vi "le fpga.vi"() -> ()   [LabVIEW 2016]
uses:
  <vilib>/LabVIEW Targets/FPGA/cRIO/shared/nicrio_ModuleControls/nicrio_cRIO-9871_BaudRateEnum.ctl
  <vilib>/LabVIEW Targets/FPGA/cRIO/shared/nicrio_ModuleControls/nicrio_cRIO-9871_ParityEnum.ctl
  <vilib>/LabVIEW Targets/FPGA/cRIO/shared/nicrio_ModuleControls/nicrio_cRIO-9871_StopBitsEnum.ctl
  <vilib>/LabVIEW Targets/FPGA/cRIO/shared/nicrio_ModuleControls/nicrio_cRIO-9871_DataBitsEnum.ctl
  <vilib>/Platform/TimedLoop/XDataNode/timing_clust.ctl
  <vilib>/Platform/TimedLoop/XDataNode/nitl_modes.ctl
  <vilib>/Platform/TimedLoop/XDataNode/wakeup.ctl
  <vilib>/rvi/FXPMathLib/basic elements/FxpIntAccumulator/subVIs/nifxpmath_IntAccumulator_SimConfig.ctl
  <vilib>/rvi/Emulation/niFpgaGetClockAttributes.vi
  <vilib>/rvi/Emulation/niFpgaSctlEmulationGetInTimedLoop.vi
  <vilib>/rvi/Emulation/niFpgaEmulationReportErrorSimple.vi
  <vilib>/rvi/eio/common/nirviEmuTemplateMethod_errors.vi
  <vilib>/rvi/Emulation/niFpgaCriticalErrorInLSC.vi
  <vilib>/rvi/Analysis/common/codeGenErrors/XNode/niFpgaXNodeCodeGenErrorHandle.vi
  <vilib>/rvi/FXPMathLib/basic elements/FxpIntAccumulator/simVIs/DllFxpIntAccumulator_sub.vi
  <vilib>/rvi/eio/common/nirviEmuTemplatePropertySet_noerrors.vi
  <vilib>/eio/EIONode/EIONode.xnode
  <vilib>/eio/EIOMethodNode/EIOMethodNode.xnode
  <vilib>/rvi/Analysis/measure/dc-rms/XNode/niFpgaDC-RMS.xnode
  <vilib>/Platform/TimedLoop/XDataNode/XDataNode.xnode
  <vilib>/rvi/FXPMathLib/basic elements/FxpIntAccumulator/XNode/nifxpmath_IntAccumulator.xnode
  <vilib>/rvi/FXPMathLib/FxpMul/XNode/nifxpmath_Multiplier.xnode
  <vilib>/eio/EIOPropertyNode/EIOPropertyNode.xnode
  <vilib>/Platform/TimedLoop/XDataNode/XDNodeRunTimeDep.lvlib
  <vilib>/rvi/FXPMathLib/sim/FxpSim.dll
  <vilib>/rvi/eio/common/nirviEmuTemplatePropertyGet_errors.vi
  <vilib>/rvi/eio/common/nirviEmuTemplatePropertyGet_noerrors.vi
  <vilib>/rvi/eio/common/nirviEmuTemplatePropertySet_errors.vi
panel:
  out "Time since repurge":u8[](array[numeric])
  out "1st stage temp(k)":u8[](array[numeric])
  out "2nd stage":u8[](array[numeric])
  out "Time on":u8[](array[numeric])
  out "Pump On":u8[](array[numeric])
  out "Ion gauge 6":u8[](array[numeric])
  out "Convectron 6":u8[](array[numeric])
  out "Convectron 5":u8[](array[numeric])
  out "Ion gauge 5":u8[](array[numeric])
  out "Analog input  2":fxp<+/-,26,5>[](array[numeric]) format="%.23g"
  in  "analog output 2":fxp<+/-,64,32>[](array[numeric])=[0.0, 0.0, 0.0, 0.0, 0.0, 0.0, 0.0]
  out "Digital readback":bool[](array[boolean])
  in  "inj image ap":bool
  in  "LE waist ap":bool
  in  "LE Waist FC":bool
  in  "ATTEN":bool
  in  "inj image  FC":bool
  in  "LE FC":bool
  out "Ion gauge 4":u8[](array[numeric])
  out "Convectron 4":u8[](array[numeric])
  out "Convectron 3":u8[](array[numeric])
  out "Ion gauge 3":u8[](array[numeric])
  in  "analog output":fxp<+/-,64,32>[](array[numeric])=[0.0, 0.0, 0.0, 0.0, 0.0, 0.0, 0.0]
  out "Analog input":fxp<+/-,26,5>[](array[numeric]) format="%.23g"
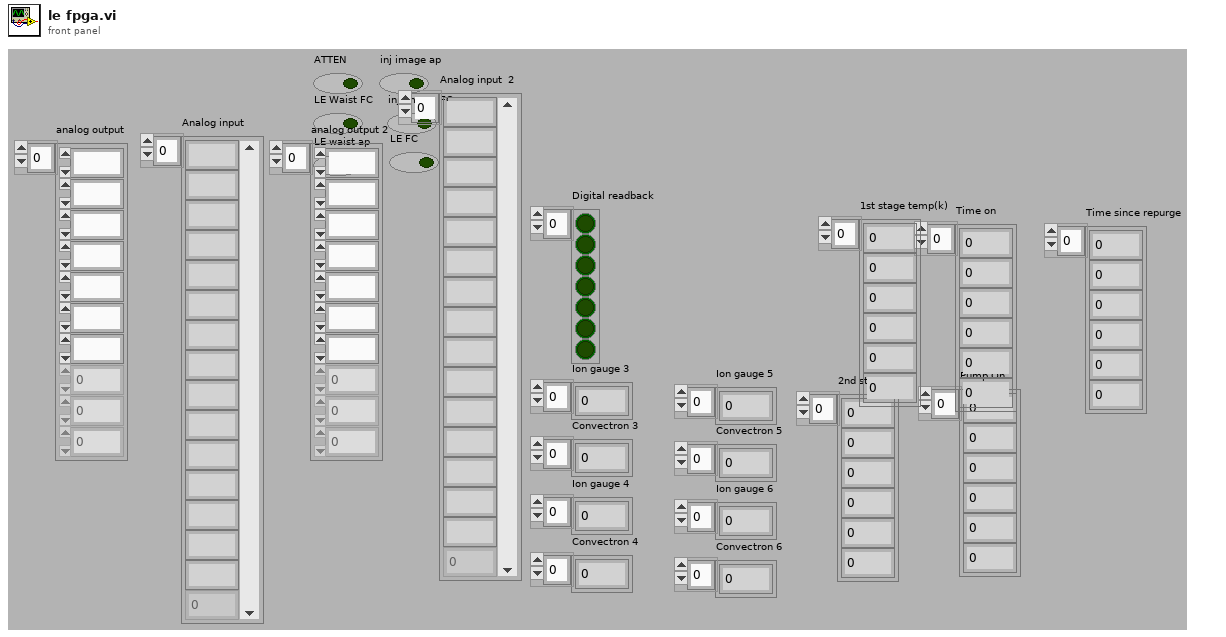
[diagram p1: front panel]
types:
  T1 = typedef "nicrio_cRIO-9871_StopBitsEnum.ctl" = enum8{"1", "1.5", "2"}
  T2 = typedef "nicrio_cRIO-9871_ParityEnum.ctl" = enum8{"None", "Odd", "Even", "Mark", "Space"}
  T3 = typedef "nicrio_cRIO-9871_DataBitsEnum.ctl" = enum8{"5", "6", "7", "8"}
  T4 = typedef "nicrio_cRIO-9871_BaudRateEnum.ctl" = enum16{"75 bps", "110 bps", "134 bps", "150 bps", "300 bps", "600 bps", "1200 bps", "1800 bps", "2400 bps", "4800 bps", "7200 bps", "9600 bps", "14.4 kbps", "19.2 kbps", "28.8 kbps", "38.4 kbps", "57.6 kbps", "115.2 kbps", "230.4 kbps", "460.8 kbps", "921.6 kbps"}
  T5 = typedef "XDNodeRunTimeDep.lvlib/timing_clust.ctl" = cluster{"Expected End [f-1]":u64, "Actual End [f-1]":u64, "Finished Late? [f-1]":bool, "Expected End [i-1]":u64, "Actual End [i-1]":u64, "Finished Late? [i-1]":bool, "Expected Start [i]":u64, "Actual Start [i]":u64, "Expected Start [f]":u64, "Actual Start [f]":u64, "Source Name":string, "Structure Name":string, "Period":i64, "Deadline":i64, "Offset":i64, "Start":i64, "Priority":i32, "Timeout":i32, "Mode":T6, "Wakeup Reason":T7, "Error":errorcluster, "Source Type":string, "Secondary Source Type":string, "Global End Time":u64, "Global Start Time":u64, "Frame Duration":u64, "Iteration Duration":u64, "Assigned CPU":i32, "I/O Scan Engine Mode":u32}
  T6 = typedef "XDNodeRunTimeDep.lvlib/nitl_modes.ctl" = enum32{"No Change", "Process missed periods, maintain original phase", "Discard missed periods, maintain original phase", "Process missed periods, ignore original phase", "Discard missed periods, ignore original phase"}
  T7 = typedef "XDNodeRunTimeDep.lvlib/wakeup.ctl" = enum32{"Normal", "Aborted", "Asynchronous wakeup", "Timing source error", "Timed loop error", "Timeout"}
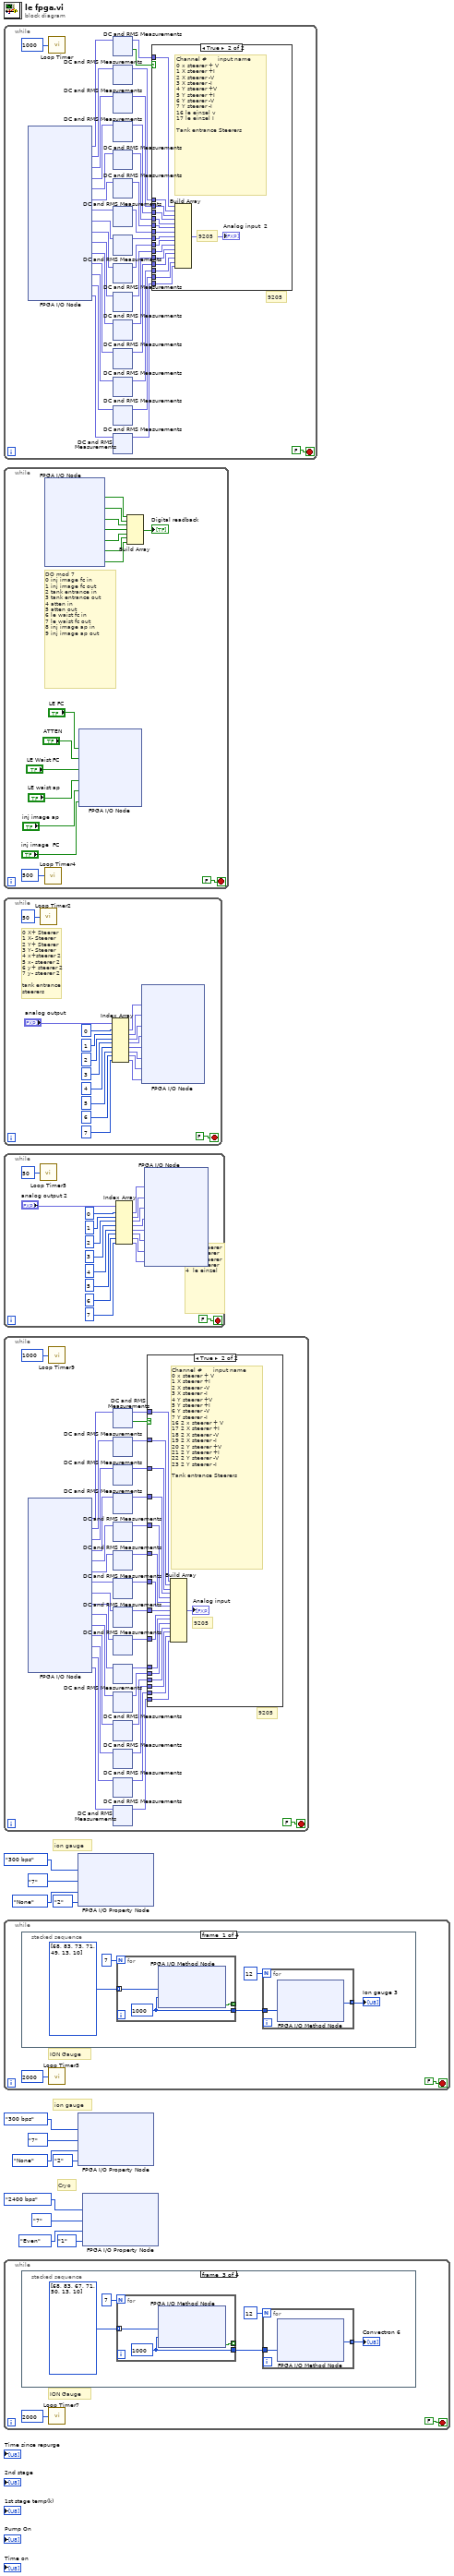
[diagram p0: block diagram]
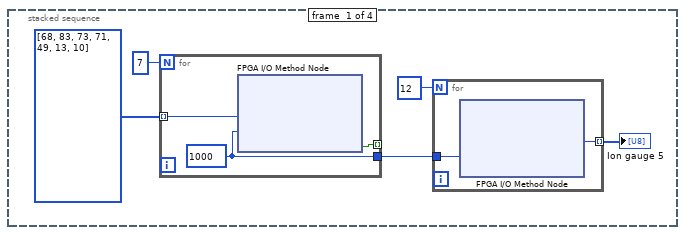
[diagram p4: hidden frame]
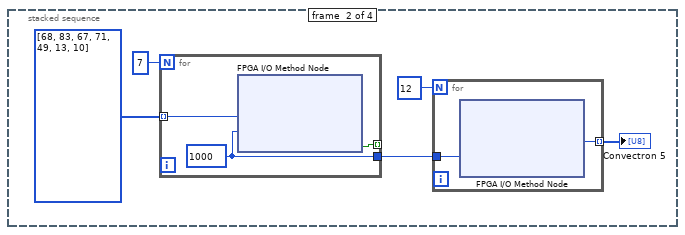
[diagram p5: hidden frame]
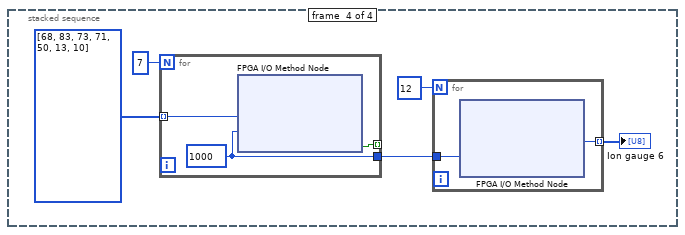
[diagram p6: hidden frame]
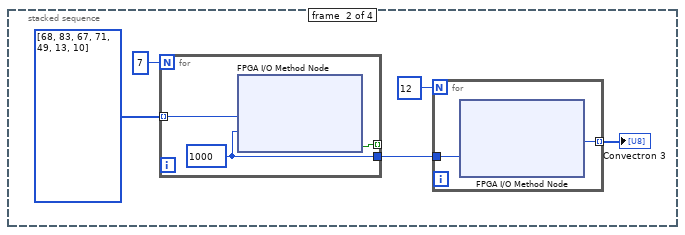
[diagram p7: hidden frame]
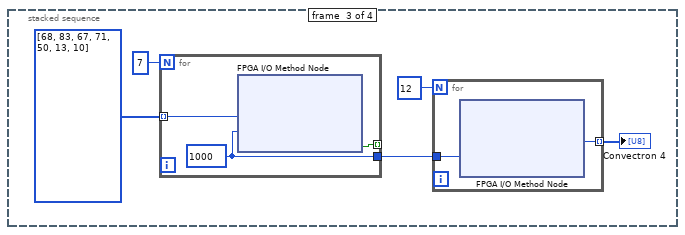
[diagram p8: hidden frame]
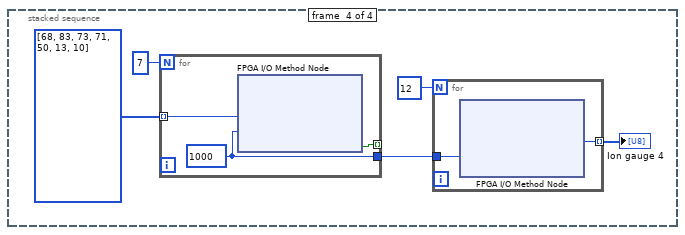
[diagram p9: hidden frame]
diagram:
  # "Cryo"
  # "ion gauge"
  # "ion gauge"
  n1 = while {
    stop <- FALSE stop-if-true
    # "9205"
    n2 = xnode "FPGA I/O Node"() -> ("Mod5/AI0"=w42:fxp<+/-,26,5>, "Mod5/AI1"=w40:fxp<+/-,26,5>, "Mod5/AI2"=w38:fxp<+/-,26,5>, "Mod5/AI3"=w36:fxp<+/-,26,5>, "Mod5/AI4"=w34:fxp<+/-,26,5>, "Mod5/AI5"=w32:fxp<+/-,26,5>, "Mod5/AI6"=w30:fxp<+/-,26,5>, "Mod5/AI7"=w28:fxp<+/-,26,5>, "Mod5/AI16"=w26:fxp<+/-,26,5>, "Mod5/AI17"=w24:fxp<+/-,26,5>, "Mod5/AI18"=w22:fxp<+/-,26,5>, "Mod5/AI19"=w20:fxp<+/-,26,5>, "Mod5/AI20"=w18:fxp<+/-,26,5>, "Mod5/AI21"=w16:fxp<+/-,26,5>, "Mod5/AI22"=w14:fxp<+/-,26,5>)  [unwired: 15 in, 15 out]
    n3 = call "Loop Timer"("Count(Ticks)"=u32 1000) -> ()  [unwired: 1 out]
    n4 = xnode "DC and RMS Measurements"("input data"=w42) -> ("DC"=w41:fxp<+/-,26,5>, "output valid"=w43:bool)  [unwired: 1 in]
    n5 = xnode "DC and RMS Measurements"("input data"=w40) -> ("DC"=w39:fxp<+/-,26,5>)  [unwired: 1 in, 1 out]
    n6 = xnode "DC and RMS Measurements"("input data"=w38) -> ("DC"=w37:fxp<+/-,26,5>)  [unwired: 1 in, 1 out]
    n7 = xnode "DC and RMS Measurements"("input data"=w36) -> ("DC"=w35:fxp<+/-,26,5>)  [unwired: 1 in, 1 out]
    n8 = xnode "DC and RMS Measurements"("input data"=w34) -> ("DC"=w33:fxp<+/-,26,5>)  [unwired: 1 in, 1 out]
    n9 = xnode "DC and RMS Measurements"("input data"=w32) -> ("DC"=w31:fxp<+/-,26,5>)  [unwired: 1 in, 1 out]
    n10 = xnode "DC and RMS Measurements"("input data"=w30) -> ("DC"=w29:fxp<+/-,26,5>)  [unwired: 1 in, 1 out]
    n11 = xnode "DC and RMS Measurements"("input data"=w28) -> ("DC"=w27:fxp<+/-,26,5>)  [unwired: 1 in, 1 out]
    n12 = xnode "DC and RMS Measurements"("input data"=w26) -> ("DC"=w25:fxp<+/-,26,5>)  [unwired: 1 in, 1 out]
    n13 = xnode "DC and RMS Measurements"("input data"=w24) -> ("DC"=w23:fxp<+/-,26,5>)  [unwired: 1 in, 1 out]
    n14 = xnode "DC and RMS Measurements"("input data"=w22) -> ("DC"=w21:fxp<+/-,26,5>)  [unwired: 1 in, 1 out]
    n15 = xnode "DC and RMS Measurements"("input data"=w20) -> ("DC"=w19:fxp<+/-,26,5>)  [unwired: 1 in, 1 out]
    n16 = xnode "DC and RMS Measurements"("input data"=w18) -> ("DC"=w17:fxp<+/-,26,5>)  [unwired: 1 in, 1 out]
    n17 = xnode "DC and RMS Measurements"("input data"=w16) -> ("DC"=w15:fxp<+/-,26,5>)  [unwired: 1 in, 1 out]
    n18 = xnode "DC and RMS Measurements"("input data"=w14) -> ("DC"=w13:fxp<+/-,26,5>)  [unwired: 1 in, 1 out]
    n19 = case shown="True" w43 {
      tunnel: w41 -> [_ w221]
      tunnel: w39 -> [_ w220]
      tunnel: w37 -> [_ w219]
      tunnel: w35 -> [_ w218]
      tunnel: w33 -> [_ w217]
      tunnel: w31 -> [_ w216]
      tunnel: w29 -> [_ w215]
      tunnel: w27 -> [_ w214]
      tunnel: w25 -> [_ w213]
      tunnel: w23 -> [_ w212]
      tunnel: w21 -> [_ w211]
      tunnel: w19 -> [_ w210]
      tunnel: w17 -> [_ w209]
      tunnel: w15 -> [_ w208]
      tunnel: w13 -> [_ w207]
      frame False {
      }
      frame True {
        # "Channel #      input name\n0 x steerer + V\n1 X steerer +I\n2 X steerer -V\n3 X steerer -I\n4 Y steerer +V\n5 Y steerer +I\n6 Y steerer -V\n7 Y steerer -I\n16 le einzel v\n17 le einzel I\n\nTank entrance Steerers"
        # "9205"
        n20 = Build Array(w221, w220, w219, w218, w217, w216, w215, w214, w213, w212, w211, w210, w209, w208, w207) -> (→"Analog input  2":fxp<+/-,26,5>[])
      }
    }
  }
  n21 = while {
    stop <- FALSE stop-if-true
    # "DO mod 7\n0 inj image fc in\n1 inj image fc out\n2 tank entrance in\n3 tank entrance out\n4 atten in\n5 atten out\n6 le waist fc in\n7 le waist fc out\n8 inj image ap in\n9 inj image ap out"
    n22 = xnode "FPGA I/O Node"() -> ("Mod7/DI0"=w1270:bool, "Mod7/DI1"=w1269:bool, "Mod7/DI2"=w1268:bool, "Mod7/DI3"=w1267:bool, "Mod7/DI4"=w1266:bool, "Mod7/DI5"=w1265:bool, "Mod7/DI6"=w1264:bool)  [unwired: 7 in, 7 out]
    n23 = call "Loop Timer4"("Count(Ticks)"=u32 500) -> ()  [unwired: 1 out]
    n24 = xnode "FPGA I/O Node"("Mod8/CH2"="LE FC", "Mod8/CH3"="ATTEN", "Mod8/CH4"="LE Waist FC", "Mod8/CH5"="LE waist ap", "Mod8/CH6"="inj image ap", "Mod8/CH1"="inj image  FC") -> ()  [unwired: 6 in, 6 out]
    n25 = Build Array(w1270, w1269, w1268, w1267, w1266, w1265, w1264) -> (→"Digital readback":bool[])
  }
  n26 = while {
    stop <- FALSE stop-if-true
    # "0 X+ Steerer\n1 X- Steerer\n2 Y+ Steerer\n3 Y- Steerer\n4 x+steerer 2\n5 x- steerer 2\n6 y+ steerer 2\n7 y- steerer 2\n\ntank entrance steerers"
    n27 = call "Loop Timer2"("Count(mSec)"=u32 50) -> ()  [unwired: 1 out]
    n28 = Index Array(array="analog output", index #1=0 ("index"), index #2=1 ("index"), index #3=2 ("index"), index #4=3 ("index"), index #5=4 ("index"), index #6=5 ("index"), index #7=6 ("index"), index #8=7 ("index")) -> (element #1=w1285:fxp<+/-,64,32>, element #2=w1284:fxp<+/-,64,32>, element #3=w1283:fxp<+/-,64,32>, element #4=w1282:fxp<+/-,64,32>, element #5=w1281:fxp<+/-,64,32>, element #6=w1280:fxp<+/-,64,32>, element #7=w1279:fxp<+/-,64,32>, element #8=w1278:fxp<+/-,64,32>)
    n29 = xnode "FPGA I/O Node"("Mod1/AO0"=w1285, "Mod1/AO1"=w1284, "Mod1/AO2"=w1283, "Mod1/AO3"=w1282, "Mod1/AO4"=w1281, "Mod1/AO5"=w1280, "Mod1/AO6"=w1279, "Mod1/AO7"=w1278) -> ()  [unwired: 8 in, 8 out]
  }
  n30 = while {
    stop <- FALSE stop-if-true
    # "0 X+ Steerer\n1 X- Steerer\n2 Y+ Steerer\n3 Y- Steerer\n4  le einzel"
    n31 = call "Loop Timer5"("Count(mSec)"=u32 50) -> ()  [unwired: 1 out]
    n32 = Index Array(array="analog output 2", index #1=0 ("index"), index #2=1 ("index"), index #3=2 ("index"), index #4=3 ("index"), index #5=4 ("index"), index #6=5 ("index"), index #7=6 ("index"), index #8=7 ("index")) -> (element #1=w1304:fxp<+/-,64,32>, element #2=w1303:fxp<+/-,64,32>, element #3=w1302:fxp<+/-,64,32>, element #4=w1301:fxp<+/-,64,32>, element #5=w1300:fxp<+/-,64,32>, element #6=w1299:fxp<+/-,64,32>, element #7=w1298:fxp<+/-,64,32>, element #8=w1297:fxp<+/-,64,32>)
    n33 = xnode "FPGA I/O Node"("Mod4/AO0"=w1304, "Mod4/AO1"=w1303, "Mod4/AO2"=w1302, "Mod4/AO3"=w1301, "Mod4/AO4"=w1300, "Mod4/AO5"=w1299, "Mod4/AO6"=w1298, "Mod4/AO7"=w1297) -> ()  [unwired: 8 in, 8 out]
  }
  n34 = while {
    stop <- FALSE stop-if-true
    # "9205"
    n35 = xnode "FPGA I/O Node"() -> ("Mod2/AI0"=w1345:fxp<+/-,26,5>, "Mod2/AI1"=w1343:fxp<+/-,26,5>, "Mod2/AI2"=w1341:fxp<+/-,26,5>, "Mod2/AI3"=w1339:fxp<+/-,26,5>, "Mod2/AI4"=w1337:fxp<+/-,26,5>, "Mod2/AI5"=w1335:fxp<+/-,26,5>, "Mod2/AI6"=w1333:fxp<+/-,26,5>, "Mod2/AI7"=w1331:fxp<+/-,26,5>, "Mod2/AI16"=w1329:fxp<+/-,26,5>, "Mod2/AI17"=w1327:fxp<+/-,26,5>, "Mod2/AI18"=w1325:fxp<+/-,26,5>, "Mod2/AI19"=w1323:fxp<+/-,26,5>, "Mod2/AI20"=w1321:fxp<+/-,26,5>, "Mod2/AI21"=w1319:fxp<+/-,26,5>, "Mod2/AI22"=w1317:fxp<+/-,26,5>)  [unwired: 15 in, 15 out]
    n36 = call "Loop Timer9"("Count(Ticks)"=u32 1000) -> ()  [unwired: 1 out]
    n37 = xnode "DC and RMS Measurements"("input data"=w1345) -> ("DC"=w1344:fxp<+/-,26,5>, "output valid"=w1346:bool)  [unwired: 1 in]
    n38 = xnode "DC and RMS Measurements"("input data"=w1343) -> ("DC"=w1342:fxp<+/-,26,5>)  [unwired: 1 in, 1 out]
    n39 = xnode "DC and RMS Measurements"("input data"=w1341) -> ("DC"=w1340:fxp<+/-,26,5>)  [unwired: 1 in, 1 out]
    n40 = xnode "DC and RMS Measurements"("input data"=w1339) -> ("DC"=w1338:fxp<+/-,26,5>)  [unwired: 1 in, 1 out]
    n41 = xnode "DC and RMS Measurements"("input data"=w1337) -> ("DC"=w1336:fxp<+/-,26,5>)  [unwired: 1 in, 1 out]
    n42 = xnode "DC and RMS Measurements"("input data"=w1335) -> ("DC"=w1334:fxp<+/-,26,5>)  [unwired: 1 in, 1 out]
    n43 = xnode "DC and RMS Measurements"("input data"=w1333) -> ("DC"=w1332:fxp<+/-,26,5>)  [unwired: 1 in, 1 out]
    n44 = xnode "DC and RMS Measurements"("input data"=w1331) -> ("DC"=w1330:fxp<+/-,26,5>)  [unwired: 1 in, 1 out]
    n45 = xnode "DC and RMS Measurements"("input data"=w1329) -> ("DC"=w1328:fxp<+/-,26,5>)  [unwired: 1 in, 1 out]
    n46 = xnode "DC and RMS Measurements"("input data"=w1327) -> ("DC"=w1326:fxp<+/-,26,5>)  [unwired: 1 in, 1 out]
    n47 = xnode "DC and RMS Measurements"("input data"=w1325) -> ("DC"=w1324:fxp<+/-,26,5>)  [unwired: 1 in, 1 out]
    n48 = xnode "DC and RMS Measurements"("input data"=w1323) -> ("DC"=w1322:fxp<+/-,26,5>)  [unwired: 1 in, 1 out]
    n49 = xnode "DC and RMS Measurements"("input data"=w1321) -> ("DC"=w1320:fxp<+/-,26,5>)  [unwired: 1 in, 1 out]
    n50 = xnode "DC and RMS Measurements"("input data"=w1319) -> ("DC"=w1318:fxp<+/-,26,5>)  [unwired: 1 in, 1 out]
    n51 = xnode "DC and RMS Measurements"("input data"=w1317) -> ("DC"=w1316:fxp<+/-,26,5>)  [unwired: 1 in, 1 out]
    n52 = case shown="True" w1346 {
      tunnel: w1344 -> [_ w1524]
      tunnel: w1342 -> [_ w1523]
      tunnel: w1340 -> [_ w1522]
      tunnel: w1338 -> [_ w1521]
      tunnel: w1336 -> [_ w1520]
      tunnel: w1334 -> [_ w1519]
      tunnel: w1332 -> [_ w1518]
      tunnel: w1330 -> [_ w1517]
      tunnel: w1328 -> [_ w1516]
      tunnel: w1326 -> [_ w1515]
      tunnel: w1324 -> [_ w1514]
      tunnel: w1322 -> [_ w1513]
      tunnel: w1320 -> [_ w1512]
      tunnel: w1318 -> [_ w1511]
      tunnel: w1316 -> [_ w1510]
      frame False {
      }
      frame True {
        # "Channel #      input name\n0 x steerer + V\n1 X steerer +I\n2 X steerer -V\n3 X steerer -I\n4 Y steerer +V\n5 Y steerer +I\n6 Y steerer -V\n7 Y steerer -I\n16 2 x steerer + V\n17 2 X steerer +I\n18 2 X steerer -V\n19 2 X steerer -I\n20 2 Y steerer +V\n21 2 Y steerer +I\n22 2 Y steerer -V\n23 2 Y steerer -I\n\nTank entrance Steerers"
        # "9205"
        n53 = Build Array(w1524, w1523, w1522, w1521, w1520, w1519, w1518, w1517, w1516, w1515, w1514, w1513, w1512, w1511, w1510) -> (→"Analog input":fxp<+/-,26,5>[])
      }
    }
  }
  n54 = while {
    stop <- FALSE stop-if-true
    # "ION Gauge"
    n55 = stacked-sequence {
      frame #0 {
        n56 = for {
          N: 7 -> [_]
          tunnel: [w2576] -> w2571
          tunnel: [w2575] -> _ mode=indexing
          tunnel: u8[] [68, 83, 73, 71, 49, 13, 10] ("unsigned byte array") -> [w2574] mode=indexing
          w2576 = 1000 ("Timeout (ms)")
          n57 = xnode "FPGA I/O Method Node"("Data"=w2574, "Timeout (ms)"=w2576) -> ("Timed Out"=w2575:bool)  [unwired: 1 in, 1 out]
        }
        n58 = for {
          N: 12 -> [_]
          tunnel: w2571 -> [w2573]
          tunnel: [w2572] -> w2567 mode=indexing
          n59 = xnode "FPGA I/O Method Node"("Timeout (ms)"=w2573) -> ("Data"=w2572:u8)  [unwired: 1 in, 2 out]
        }
        "Ion gauge 3" <- w2567
      }
      frame #1 {
        n60 = for {
          N: 7 -> [_]
          tunnel: [w2586] -> w2581
          tunnel: [w2585] -> _ mode=indexing
          tunnel: u8[] [68, 83, 67, 71, 49, 13, 10] ("unsigned byte array") -> [w2584] mode=indexing
          w2586 = 1000 ("Timeout (ms)")
          n61 = xnode "FPGA I/O Method Node"("Data"=w2584, "Timeout (ms)"=w2586) -> ("Timed Out"=w2585:bool)  [unwired: 1 in, 1 out]
        }
        n62 = for {
          N: 12 -> [_]
          tunnel: w2581 -> [w2583]
          tunnel: [w2582] -> w2577 mode=indexing
          n63 = xnode "FPGA I/O Method Node"("Timeout (ms)"=w2583) -> ("Data"=w2582:u8)  [unwired: 1 in, 2 out]
        }
        "Convectron 3" <- w2577
      }
      frame #2 {
        n64 = for {
          N: 7 -> [_]
          tunnel: [w2596] -> w2591
          tunnel: [w2595] -> _ mode=indexing
          tunnel: u8[] [68, 83, 67, 71, 50, 13, 10] ("unsigned byte array") -> [w2594] mode=indexing
          w2596 = 1000 ("Timeout (ms)")
          n65 = xnode "FPGA I/O Method Node"("Data"=w2594, "Timeout (ms)"=w2596) -> ("Timed Out"=w2595:bool)  [unwired: 1 in, 1 out]
        }
        n66 = for {
          N: 12 -> [_]
          tunnel: w2591 -> [w2593]
          tunnel: [w2592] -> w2587 mode=indexing
          n67 = xnode "FPGA I/O Method Node"("Timeout (ms)"=w2593) -> ("Data"=w2592:u8)  [unwired: 1 in, 2 out]
        }
        "Convectron 4" <- w2587
      }
      frame #3 {
        n68 = for {
          N: 7 -> [_]
          tunnel: [w2606] -> w2601
          tunnel: [w2605] -> _ mode=indexing
          tunnel: u8[] [68, 83, 73, 71, 50, 13, 10] ("unsigned byte array") -> [w2604] mode=indexing
          w2606 = 1000 ("Timeout (ms)")
          n69 = xnode "FPGA I/O Method Node"("Data"=w2604, "Timeout (ms)"=w2606) -> ("Timed Out"=w2605:bool)  [unwired: 1 in, 1 out]
        }
        n70 = for {
          N: 12 -> [_]
          tunnel: w2601 -> [w2603]
          tunnel: [w2602] -> w2597 mode=indexing
          n71 = xnode "FPGA I/O Method Node"("Timeout (ms)"=w2603) -> ("Data"=w2602:u8)  [unwired: 1 in, 2 out]
        }
        "Ion gauge 4" <- w2597
      }
    }
    n72 = call "Loop Timer3"("Count(mSec)"=u32 2000 ("Count(Ticks)")) -> ()  [unwired: 1 out]
  }
  n73 = while {
    stop <- FALSE stop-if-true
    # "ION Gauge"
    n74 = stacked-sequence {
      frame #0 {
        n75 = for {
          N: 7 -> [_]
          tunnel: [w2618] -> w2613
          tunnel: [w2617] -> _ mode=indexing
          tunnel: u8[] [68, 83, 73, 71, 49, 13, 10] ("unsigned byte array") -> [w2616] mode=indexing
          w2618 = 1000 ("Timeout (ms)")
          n76 = xnode "FPGA I/O Method Node"("Data"=w2616, "Timeout (ms)"=w2618) -> ("Timed Out"=w2617:bool)  [unwired: 1 in, 1 out]
        }
        n77 = for {
          N: 12 -> [_]
          tunnel: w2613 -> [w2615]
          tunnel: [w2614] -> w2609 mode=indexing
          n78 = xnode "FPGA I/O Method Node"("Timeout (ms)"=w2615) -> ("Data"=w2614:u8)  [unwired: 1 in, 2 out]
        }
        "Ion gauge 5" <- w2609
      }
      frame #1 {
        n79 = for {
          N: 7 -> [_]
          tunnel: [w2628] -> w2623
          tunnel: [w2627] -> _ mode=indexing
          tunnel: u8[] [68, 83, 67, 71, 49, 13, 10] ("unsigned byte array") -> [w2626] mode=indexing
          w2628 = 1000 ("Timeout (ms)")
          n80 = xnode "FPGA I/O Method Node"("Data"=w2626, "Timeout (ms)"=w2628) -> ("Timed Out"=w2627:bool)  [unwired: 1 in, 1 out]
        }
        n81 = for {
          N: 12 -> [_]
          tunnel: w2623 -> [w2625]
          tunnel: [w2624] -> w2619 mode=indexing
          n82 = xnode "FPGA I/O Method Node"("Timeout (ms)"=w2625) -> ("Data"=w2624:u8)  [unwired: 1 in, 2 out]
        }
        "Convectron 5" <- w2619
      }
      frame #2 {
        n83 = for {
          N: 7 -> [_]
          tunnel: [w2638] -> w2633
          tunnel: [w2637] -> _ mode=indexing
          tunnel: u8[] [68, 83, 67, 71, 50, 13, 10] ("unsigned byte array") -> [w2636] mode=indexing
          w2638 = 1000 ("Timeout (ms)")
          n84 = xnode "FPGA I/O Method Node"("Data"=w2636, "Timeout (ms)"=w2638) -> ("Timed Out"=w2637:bool)  [unwired: 1 in, 1 out]
        }
        n85 = for {
          N: 12 -> [_]
          tunnel: w2633 -> [w2635]
          tunnel: [w2634] -> w2629 mode=indexing
          n86 = xnode "FPGA I/O Method Node"("Timeout (ms)"=w2635) -> ("Data"=w2634:u8)  [unwired: 1 in, 2 out]
        }
        "Convectron 6" <- w2629
      }
      frame #3 {
        n87 = for {
          N: 7 -> [_]
          tunnel: [w2648] -> w2643
          tunnel: [w2647] -> _ mode=indexing
          tunnel: u8[] [68, 83, 73, 71, 50, 13, 10] ("unsigned byte array") -> [w2646] mode=indexing
          w2648 = 1000 ("Timeout (ms)")
          n88 = xnode "FPGA I/O Method Node"("Data"=w2646, "Timeout (ms)"=w2648) -> ("Timed Out"=w2647:bool)  [unwired: 1 in, 1 out]
        }
        n89 = for {
          N: 12 -> [_]
          tunnel: w2643 -> [w2645]
          tunnel: [w2644] -> w2639 mode=indexing
          n90 = xnode "FPGA I/O Method Node"("Timeout (ms)"=w2645) -> ("Data"=w2644:u8)  [unwired: 1 in, 2 out]
        }
        "Ion gauge 6" <- w2639
      }
    }
    n91 = call "Loop Timer7"("Count(mSec)"=u32 2000 ("Count(Ticks)")) -> ()  [unwired: 1 out]
  }
  n92 = xnode "FPGA I/O Property Node"("Baud Rate"=nicrio_cRIO-9871_BaudRateEnum."300 bps", "Data Bits"=nicrio_cRIO-9871_DataBitsEnum."7", "Parity"=nicrio_cRIO-9871_ParityEnum."None", "Stop Bits"=nicrio_cRIO-9871_StopBitsEnum."2") -> ()  [unwired: 1 in, 1 out]
  n93 = xnode "FPGA I/O Property Node"("Baud Rate"=nicrio_cRIO-9871_BaudRateEnum."300 bps", "Data Bits"=nicrio_cRIO-9871_DataBitsEnum."7", "Parity"=nicrio_cRIO-9871_ParityEnum."None", "Stop Bits"=nicrio_cRIO-9871_StopBitsEnum."2") -> ()  [unwired: 1 in, 1 out]
  n94 = xnode "FPGA I/O Property Node"("Baud Rate"=nicrio_cRIO-9871_BaudRateEnum."2400 bps", "Data Bits"=nicrio_cRIO-9871_DataBitsEnum."7", "Parity"=nicrio_cRIO-9871_ParityEnum."Even", "Stop Bits"=nicrio_cRIO-9871_StopBitsEnum."1") -> ()  [unwired: 1 in, 1 out]
